vi "Save Encoder Data From MyRio.vi"() -> ()   [LabVIEW 2018]
panel:
  out "Output String":string
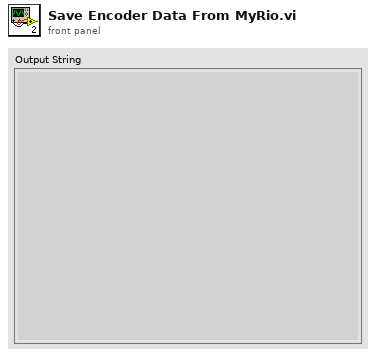
[diagram p1: front panel]
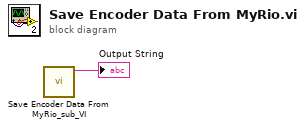
[diagram p0: block diagram]
diagram:
  n1 = call "Save Encoder Data From MyRio_sub_VI.vi"() -> ("Output String"=→"Output String":string)  [unwired: 11 in]
